vi "Test.vi"() -> ()   [LabVIEW 2018]
uses:
  controls/openModbusConnectionCluster.ctl
  controls/writeSingleRegisterModbusCluster.ctl
  controls/modbusDriverSelectorEnum.ctl
  controls/readRegisterModbusCluster.ctl
panel:
  in  "Register to write":u16
  in  "Address":u16
  in  "Write":bool
  out "Boolean":bool
  in  "Port":u16=255
  in  "Timeout":i32=500
  in  "IP Address":string
  in  "OK":bool
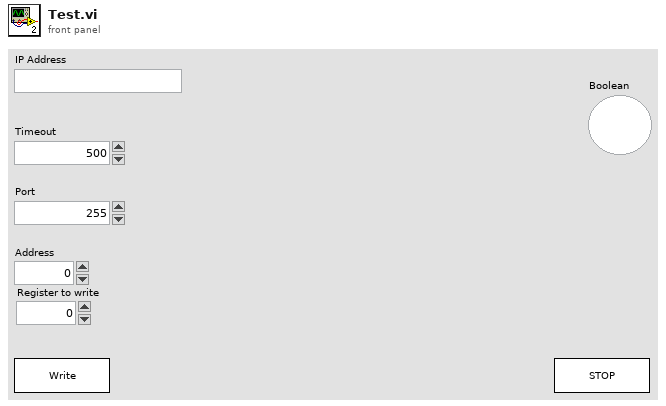
[diagram p1: front panel]
types:
  T1 = enum32{"Invalid", "Standard", "Closed", "Hidden", "Minimized", "Maximized"}
  T2 = enum32{"invalid app kind", "Development System", "Run Time System", "Student Edition", "Embedded LabVIEW", "Evaluation", "Custom"}
  T3 = typedef "writeSingleRegisterModbusCluster.ctl" = cluster{"Address":u16, "Register to write":u16}
  T4 = typedef "openModbusConnectionCluster.ctl" = cluster{"IP Address":string, "Timeout (ms)":i32, "Port (502)":u16}
  T5 = typedef "modbusDriverSelectorEnum.ctl" = enum16{"open", "write single holding registers", "read holding registers", "close"}
  T6 = typedef "readRegisterModbusCluster.ctl" = cluster{"Starting Address":u16, "Number of Inputs":u16}
  T7 = cluster{"Core":cluster{"Current VI Reference":refnum<vi>, "Close Panel on Exit?":bool}, "Open Modbus Connection Cluster":T4, bool, "Write Single Register Modbus":T3}
  T8 = cluster{"Current VI Reference":refnum<vi>, "Close Panel on Exit?":bool}
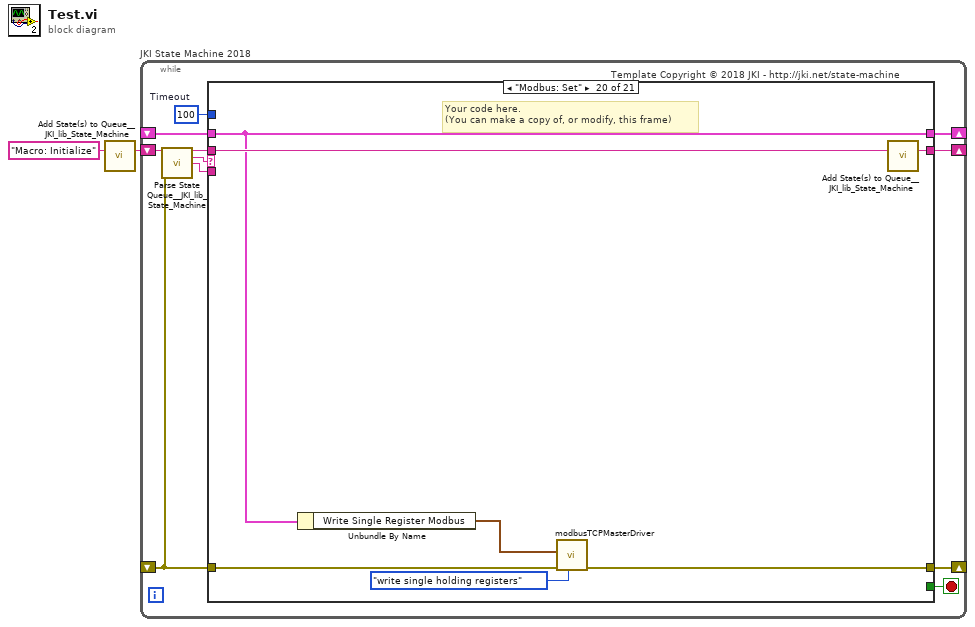
[diagram p0: block diagram]
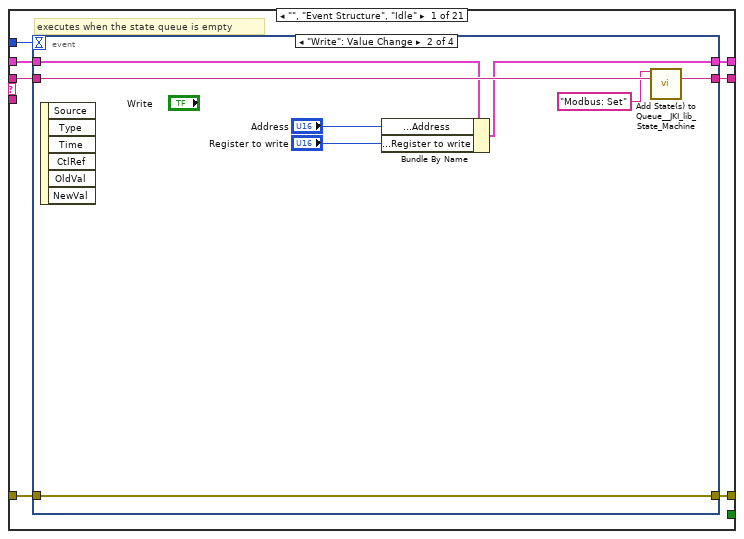
[diagram p2: hidden frame]
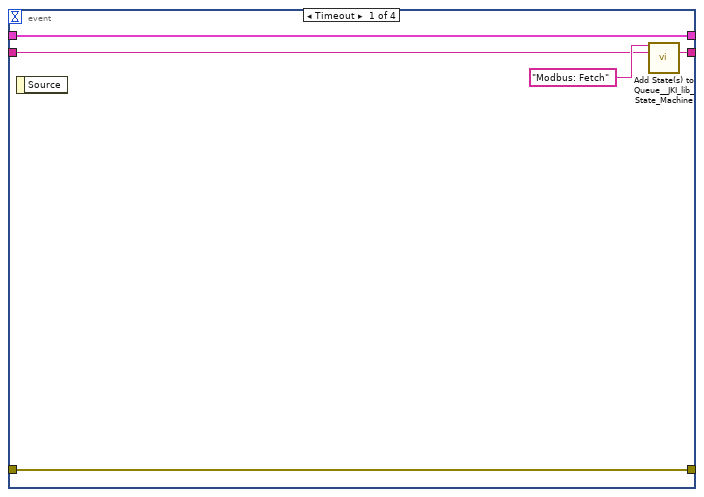
[diagram p3: hidden frame]
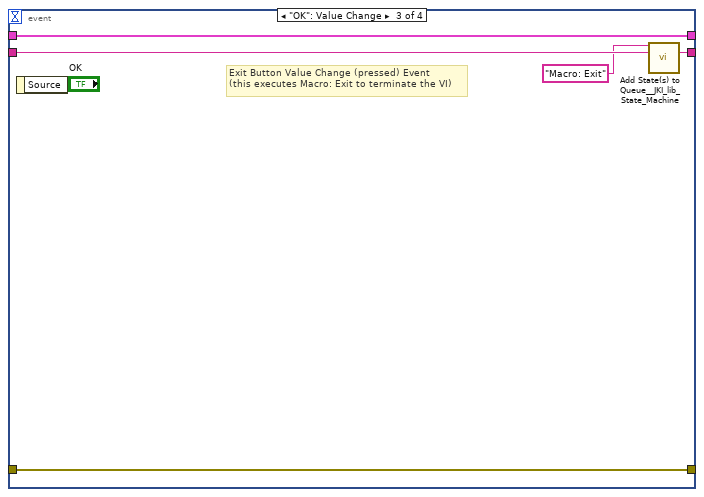
[diagram p4: hidden frame]
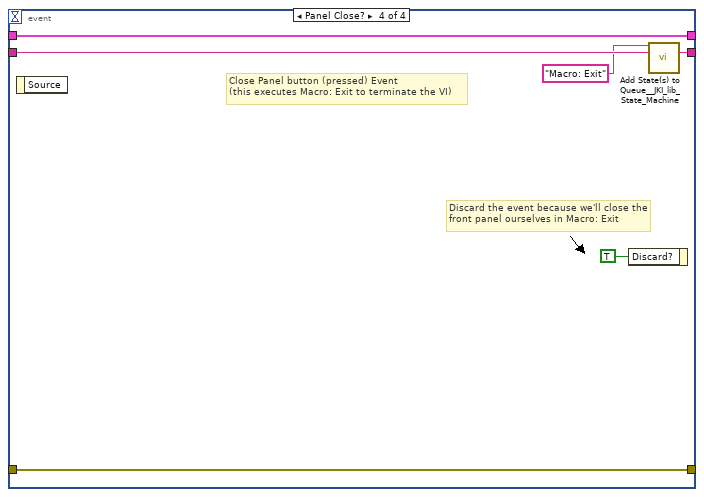
[diagram p5: hidden frame]
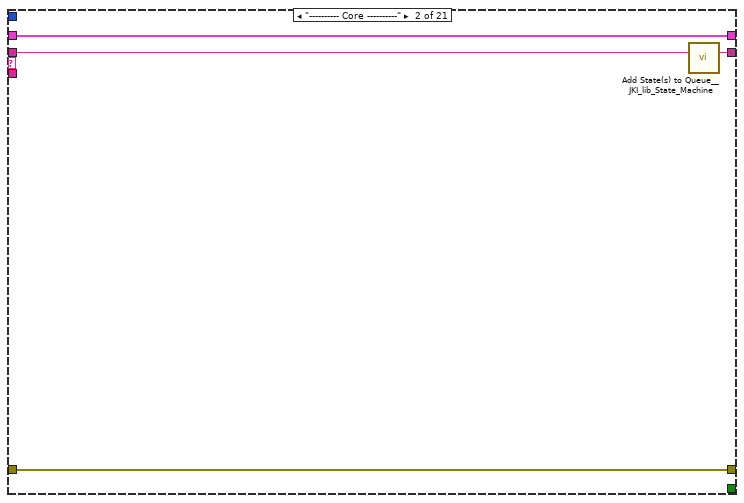
[diagram p6: hidden frame]
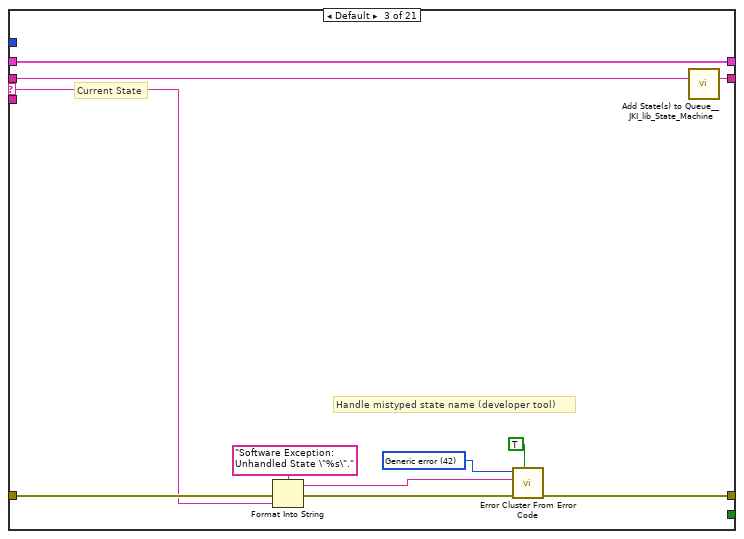
[diagram p7: hidden frame]
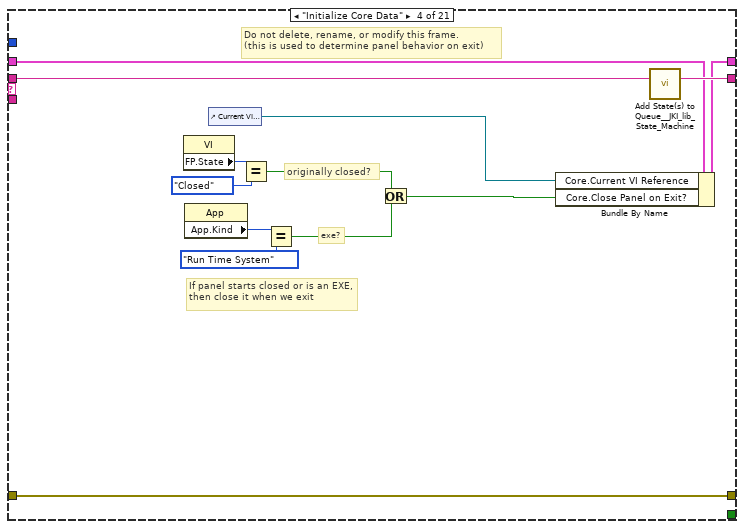
[diagram p8: hidden frame]
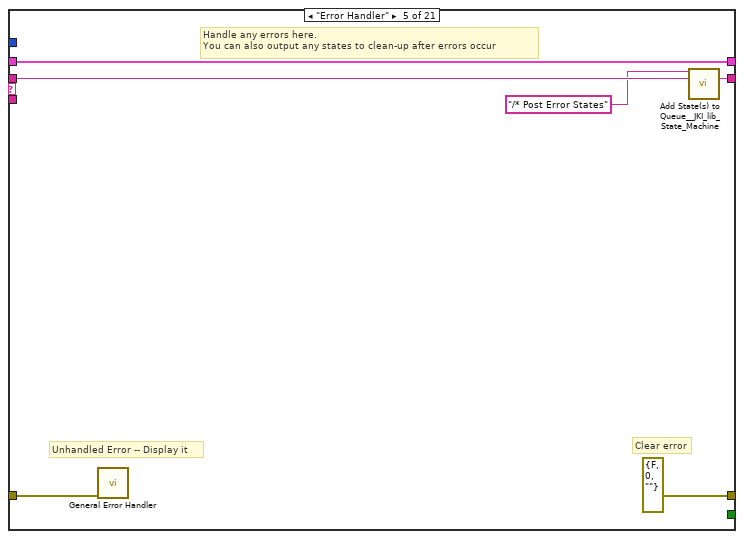
[diagram p9: hidden frame]
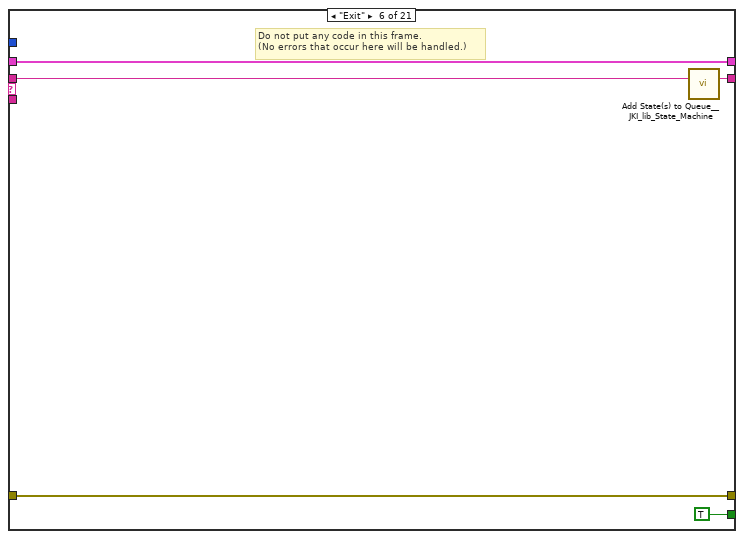
[diagram p10: hidden frame]
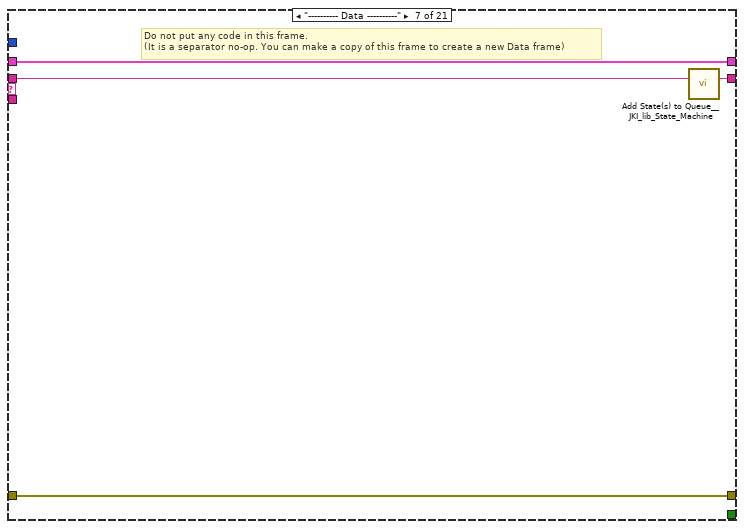
[diagram p11: hidden frame]
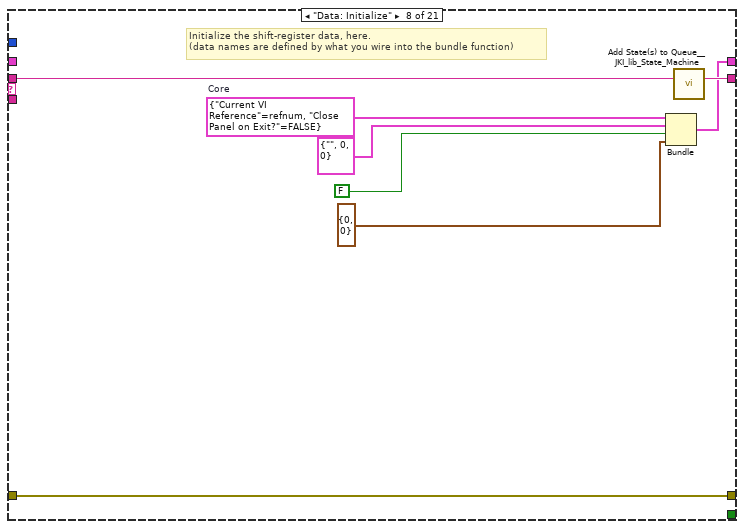
[diagram p12: hidden frame]
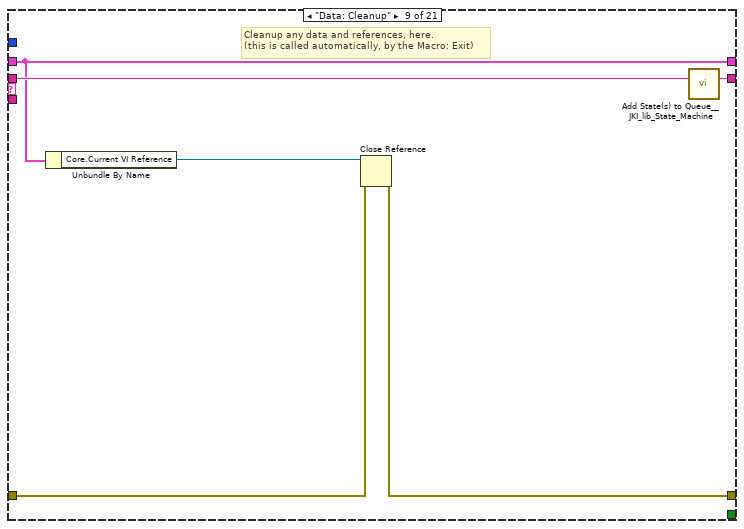
[diagram p13: hidden frame]
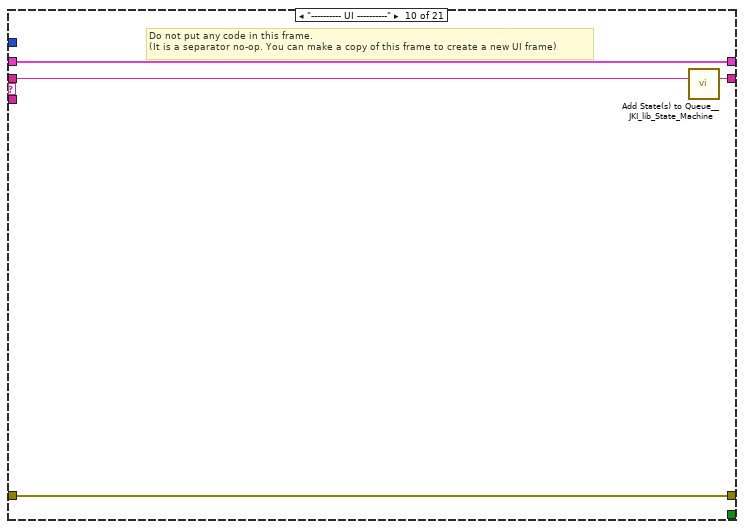
[diagram p14: hidden frame]
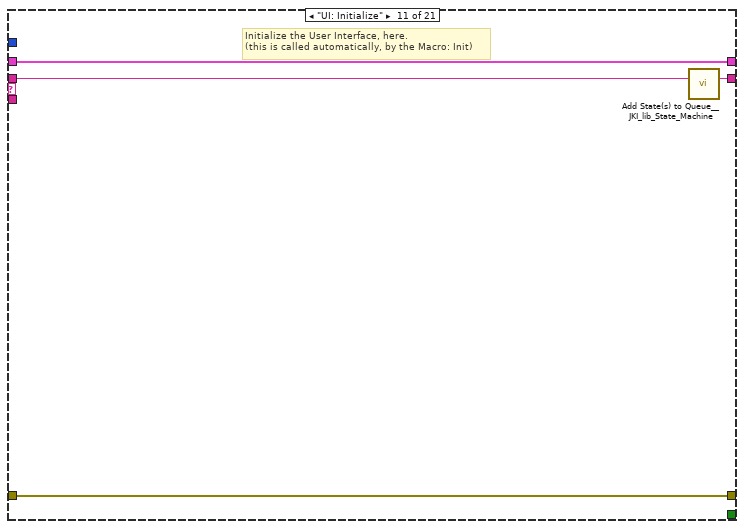
[diagram p15: hidden frame]
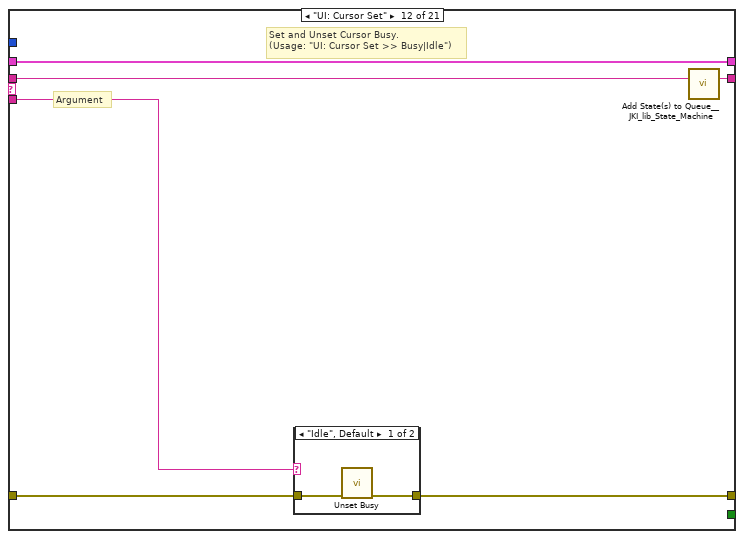
[diagram p16: hidden frame]
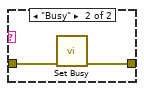
[diagram p17: hidden frame]
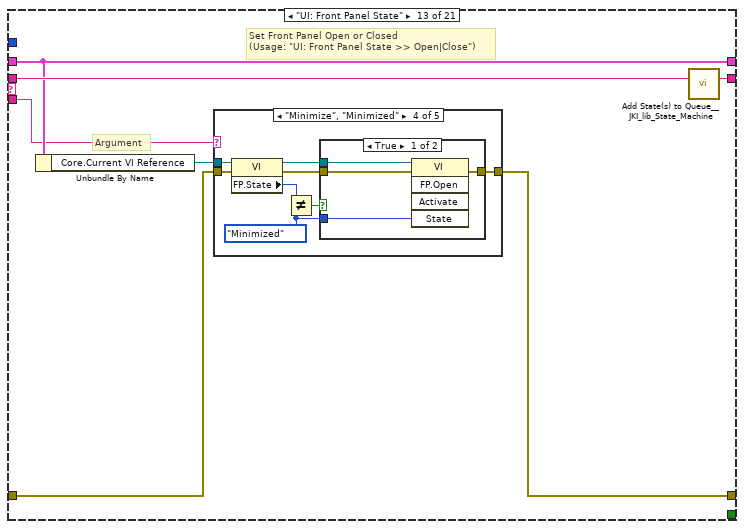
[diagram p18: hidden frame]
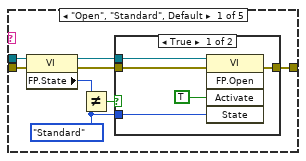
[diagram p19: hidden frame]
diagram:
  n1 = call <vilib>:"Add State(s) to Queue__JKI_lib_State_Machine.vi"("State(s) in (\"\")"="Macro: Initialize") -> ("States Out"=w2:string)  [unwired: 14 in]
  n2 = while "JKI State Machine 2018" {
    shift-right: [w6] -> _
    shift-left: _ -> [w5]
    shift-right: [w9] -> _
    shift-left: _ -> [w3]
    shift-right: [w8] -> _
    shift-left: w2 -> [w10]
    stop <- w7 stop-if-true
    w4 = 100  # Timeout
    # "Template Copyright © 2018 JKI - http://jki.net/state-machine"
    n3 = call <vilib>:"Parse State Queue__JKI_lib_State_Machine.vi"("State Queue"=w10, "Error In (no error)"=w3) -> ("Remaining States"=w12:string, "Current State"=w13:string, "Arguments"=w11:string)  [unwired: 11 in]
    n4 = case shown="\"Modbus: Set\"" w13 {
      selector: w13 -> [_ _ w49 _ _ _ _ _ _ _ _ _ _ _ _ _ _ _ _ _ _]
      tunnel: w12 -> [w20 w48 w53 w72 w78 w83 w87 w95 w101 w105 w109 w115 w126 w195 w200 w210 w214 w225 w239 w249 w253]
      tunnel: w11 -> [_ _ _ _ _ _ _ _ _ _ _ w110 w120 _ _ _ _ _ _ _ _]
      tunnel: w5 -> [w18 w45 w51 w65 w75 w81 w84 _ w96 w102 w107 w113 w122 w192 w197 w207 w211 w223 w237 w244 w250]
      tunnel: [w17 w46 w55 w69 errorcluster {"status"=FALSE, "code"=0, "source"=""} ("error out") w80 w85 w92 w97 w103 w106 w111 w123 w193 w198 w208 w212 w221 w235 w246 w251] -> w9
      tunnel: w3 -> [w16 w46 w54 w69 w74 w80 w85 w92 w98 w103 w106 w112 w124 w193 w198 w208 w212 w222 w236 w247 w251]
      tunnel: [w19 w47 w52 w71 w77 w82 w86 w94 w100 w104 w108 w114 w125 w194 w199 w209 w213 w224 w238 w248 w252] -> w8
      tunnel: [_ _ _ _ _ TRUE _ _ _ _ _ _ _ _ _ _ _ _ _ _ _] -> w7
      tunnel: [w15 w45 w51 w70 w75 w81 w84 w93 w96 w102 w107 w113 w122 w192 w197 w207 w211 w223 w237 w244 w250] -> w6
      tunnel: w4 -> [w14 _ _ _ _ _ _ _ _ _ _ _ _ _ _ _ _ _ _ _ _]
      frame "", "Event Structure", "Idle" {
        # "executes when the state queue is empty"
        n5 = event shown="[1] \"Write\": Value Change" {
          selector: _ -> [_ _ _ _]
          dyn-events: _ -> [_ _ _ _]
          timeout: w14 -> [_ _ _ _]
          tunnel: w20 -> [w21 w33 w38 w44]
          tunnel: [w25 w32 w37 w43] -> w19
          tunnel: w18 -> [w23 w30 w35 w41]
          tunnel: [w24 w27 w36 w42] -> w17
          tunnel: w16 -> [w24 w27 w36 w42]
          tunnel: [w23 w29 w35 w41] -> w15
          event Timeout {
            n6 = event-data() -> ()  [unwired: 1 in, 1 out]
            n7 = call <vilib>:"Add State(s) to Queue__JKI_lib_State_Machine.vi"("State(s) in Front (\"\")"="Modbus: Fetch", "State(s) in (\"\")"=w21) -> ("States Out"=w25:string)  [unwired: 13 in]
          }
          event "Write": Value Change {
            n8 = event-data() -> ()  [unwired: 1 in, 6 out]
            n9 = Bundle By Name(cluster=w30, "Write Single Register Modbus.Address"="Address", "Write Single Register Modbus.Register to write"="Register to write") -> (w29:T7)
            n10 = call <vilib>:"Add State(s) to Queue__JKI_lib_State_Machine.vi"("State(s) in Front (\"\")"="Modbus: Set" ("State(s) in Front (\"\")"), "State(s) in (\"\")"=w33) -> ("States Out"=w32:string)  [unwired: 13 in]
          }
          event "OK": Value Change {
            # "Exit Button Value Change (pressed) Event\n(this executes Macro: Exit to terminate the VI)"
            n11 = event-data() -> ()  [unwired: 1 in, 1 out]
            n12 = call <vilib>:"Add State(s) to Queue__JKI_lib_State_Machine.vi"("State(s) in Front (\"\")"="Macro: Exit", "State(s) in (\"\")"=w38) -> ("States Out"=w37:string)  [unwired: 13 in]
          }
          event Panel Close? {
            # "Discard the event because we'll close the front panel ourselves in Macro: Exit"
            # "Close Panel button (pressed) Event\n(this executes Macro: Exit to terminate the VI)"
            n13 = event-data() -> ()  [unwired: 1 in, 1 out]
            n14 = event-data("Discard?"=TRUE) -> ()  [unwired: 1 in, 1 out]
            n15 = call <vilib>:"Add State(s) to Queue__JKI_lib_State_Machine.vi"("State(s) in Front (\"\")"="Macro: Exit", "State(s) in (\"\")"=w44) -> ("States Out"=w43:string)  [unwired: 13 in]
          }
        }
      }
      frame "---------- Core ----------" {
        n16 = call <vilib>:"Add State(s) to Queue__JKI_lib_State_Machine.vi"("State(s) in (\"\")"=w48) -> ("States Out"=w47:string)  [unwired: 14 in]
      }
      frame Default {
        w58 = 42 items=["No error", "Argument error", "Memory is full", "Out of zone", "End of file", "File already open", "Generic file I/O error", "File not found", "File permission error", "Disk is full", "Duplicate path", "Too many files open", "System feature not enabled", "Resource file not found", "Cannot add resource", "Resource not found", "Image not found", "Image memory error", "Pen does not exist", "Config type invalid", "Config token not found", "Config parse error", "Config memory error", "Bad external code format", "Bad external code offset", "External code not present", "Null window", "Destroy window error", "Null menu", "Print aborted", "Bad print record", "Print driver error", "Windows error during printing", "Memory error during printing", "Print dialog error", "Generic print error", "Invalid device refnum", "Device not found", "Device parameter error", "Device unit error", "Cannot open device", "Device call aborted", "Generic error", "Cancelled by user", "Object ID too low", "Object ID too high", "Object not in heap", "Unknown heap", "Unknown object (invalid DefProc)", "Unknown object (DefProc not in table)", "Message out of range", "Invalid (null) method", "Unknown message", "Manager call not supported", "Bad address", "Network operation in progress", "Network operation timed out", "Connection is busy", "Network attribute not supported", "Network error", "Address in use", "System out of memory", "Connection aborted", "Connection refused", "Not connected", "Already connected", "Connection closed", "Initialization error (interapplication manager)", "Bad occurrence", "Wait on unbound occurrence handler", "Occurrence queue overflow", "Datalog type conflict", "Unused", "Unrecognized type (interapplication manager)", "Memory corrupt", "Failed to make temporary DLL", "Old CIN version", "Drag socket not found", "Failed to load drop-object", "Failed to register OLE object", "Failed to release OLE object", "Format specifier type mismatch", "Unknown format specifier", "Too few format specifiers", "Too many format specifiers", "Scan failed", "Newer CIN version", "Error converting to variant", "Runtime menu error", "Password tampered", "Variant attribute not found", "Incompatible variant data type", "Event data is not available", "Event Store is not present", "Occurrence is not found", "Event Queue is not created", "Event info is not available", "Refnum passed is NULL", "Error retrieving Class GUID", "Error retrieving CoClass GUID", "Error retrieving TypeLib GUID.", "Bad built application magic bytes.", "Specific driver is different from the specific driver associated with the Logical Name.", "There is no session opened to the class driver.", "Max Error", "MAX - Error with config objects", "MAX - Error loading configuration", "MAX - Group not supported"]
        # "Current State"
        # "Handle mistyped state name (developer tool)"
        n17 = Format Into String(format string="Software Exception: Unhandled State \"%s\"." ("message"), error in=w54, w49) -> (resulting string=w57:string, error out=w56:errorcluster)  [unwired: 1 in]
        n18 = call <vilib>:"Error Cluster From Error Code.vi"("show call chain? (False)"=TRUE, "error in (no error)"=w56, "error message (\"\")"=w57, "error code (0)"=w58) -> ("error out"=w55:errorcluster)  [unwired: 5 in]
        n19 = call <vilib>:"Add State(s) to Queue__JKI_lib_State_Machine.vi"("State(s) in (\"\")"=w53) -> ("States Out"=w52:string)  [unwired: 14 in]
      }
      frame "Initialize Core Data" {
        # "Do not delete, rename, or modify this frame.\n(this is used to determine panel behavior on exit)"
        # "originally closed?"
        # "exe?"
        # "If panel starts closed or is an EXE, then close it when we exit"
        n20 = property class="VI"() -> ("FP.State"=w62:T1)  [unwired: 2 in, 2 out]
        n21 = property class="App"() -> ("App.Kind"=w68:T2)  [unwired: 2 in, 2 out]
        n22 = control-ref of="Current VI Reference"() -> (w63:refnum<vi>)
        n23 = Equal?(x=w62, y=T1."Closed" ("Front Panel Window:State")) -> (x = y?=w60:bool)
        n24 = Equal?(x=w68, y=T2."Run Time System" ("Application:Kind")) -> (x = y?=w66:bool)
        n25 = Or(x=w60, y=w66) -> (x .or. y?=w64:bool)
        n26 = Bundle By Name(cluster=w65, "Core.Current VI Reference"=w63, "Core.Close Panel on Exit?"=w64) -> (w70:T7)
        n27 = call <vilib>:"Add State(s) to Queue__JKI_lib_State_Machine.vi"("State(s) in (\"\")"=w72) -> ("States Out"=w71:string)  [unwired: 14 in]
      }
      frame "Error Handler" {
        # "Unhandled Error -- Display it"
        # "Handle any errors here.\nYou can also output any states to clean-up after errors occur"
        # "Clear error"
        n28 = call <vilib>:"General Error Handler.vi"("error in (no error)"=w74) -> ()  [unwired: 10 in, 5 out]
        n29 = call <vilib>:"Add State(s) to Queue__JKI_lib_State_Machine.vi"("State(s) in Front (\"\")"="/* Post Error States", "State(s) in (\"\")"=w78) -> ("States Out"=w77:string)  [unwired: 13 in]
      }
      frame "Exit" {
        # "Do not put any code in this frame.\n(No errors that occur here will be handled.)"
        n30 = call <vilib>:"Add State(s) to Queue__JKI_lib_State_Machine.vi"("State(s) in (\"\")"=w83) -> ("States Out"=w82:string)  [unwired: 14 in]
      }
      frame "---------- Data ----------" {
        # "Do not put any code in this frame.\n(It is a separator no-op. You can make a copy of this frame to create a new Data frame)"
        n31 = call <vilib>:"Add State(s) to Queue__JKI_lib_State_Machine.vi"("State(s) in (\"\")"=w87) -> ("States Out"=w86:string)  [unwired: 14 in]
      }
      frame "Data: Initialize" {
        w91 = T8 {"Current VI Reference"=refnum, "Close Panel on Exit?"=FALSE}  # Core
        # "Initialize the shift-register data, here.\n(data names are defined by what you wire into the bundle function)"
        n32 = Bundle("Core"=w91, "Open Modbus Connection Cluster"=T4 {"IP Address"="", "Timeout (ms)"=0, "Port (502)"=0}, FALSE, "Write Single Register Modbus"=T3 {"Address"=0, "Register to write"=0}) -> (w93:T7)  [unwired: 1 in]
        n33 = call <vilib>:"Add State(s) to Queue__JKI_lib_State_Machine.vi"("State(s) in (\"\")"=w95) -> ("States Out"=w94:string)  [unwired: 14 in]
      }
      frame "Data: Cleanup" {
        # "Cleanup any data and references, here.\n(this is called automatically, by the Macro: Exit)"
        n34 = Unbundle By Name(w96) -> ("Core.Current VI Reference"=w99:refnum<vi>)
        n35 = Close Reference(reference=w99, error in (no error)=w98) -> (error out=w97:errorcluster)
        n36 = call <vilib>:"Add State(s) to Queue__JKI_lib_State_Machine.vi"("State(s) in (\"\")"=w101) -> ("States Out"=w100:string)  [unwired: 14 in]
      }
      frame "---------- UI ----------" {
        # "Do not put any code in this frame.\n(It is a separator no-op. You can make a copy of this frame to create a new UI frame)"
        n37 = call <vilib>:"Add State(s) to Queue__JKI_lib_State_Machine.vi"("State(s) in (\"\")"=w105) -> ("States Out"=w104:string)  [unwired: 14 in]
      }
      frame "UI: Initialize" {
        # "Initialize the User Interface, here.\n(this is called automatically, by the Macro: Init)"
        n38 = call <vilib>:"Add State(s) to Queue__JKI_lib_State_Machine.vi"("State(s) in (\"\")"=w109) -> ("States Out"=w108:string)  [unwired: 14 in]
      }
      frame "UI: Cursor Set" {
        # "Argument"
        # "Set and Unset Cursor Busy.\n(Usage: \"UI: Cursor Set >> Busy|Idle\")"
        n39 = case shown="\"Idle\", Default" w110 {
          tunnel: w112 -> [w117 w119]
          tunnel: [w116 w118] -> w111
          frame "Idle", Default {
            n40 = call <vilib>:"Unset Busy.vi"("error in (no error)"=w117) -> ("error out"=w116:errorcluster)  [unwired: 10 in]
          }
          frame "Busy" {
            n41 = call <vilib>:"Set Busy.vi"("error in (no error)"=w119) -> ("error out"=w118:errorcluster)  [unwired: 9 in, 1 out]
          }
        }
        n42 = call <vilib>:"Add State(s) to Queue__JKI_lib_State_Machine.vi"("State(s) in (\"\")"=w115) -> ("States Out"=w114:string)  [unwired: 14 in]
      }
      frame "UI: Front Panel State" {
        # "Argument"
        # "Set Front Panel Open or Closed\n(Usage: \"UI: Front Panel State >> Open|Close\")"
        n43 = Unbundle By Name(w122) -> ("Core.Current VI Reference"=w121:refnum<vi>)
        n44 = case shown="\"Minimize\", \"Minimized\"" w120 {
          tunnel: w124 -> [w132 w147 w158 w171 w184]
          tunnel: [w134 w148 w160 w173 w186] -> w123
          tunnel: w121 -> [w133 w145 w159 w172 w185]
          frame "Open", "Standard", Default {
            w127 = T1."Standard" ("State")
            n45 = property class="VI"(reference=w133, error in=w132) -> (reference out=w130:refnum<vi>, error out=w131:errorcluster, "FP.State"=w129:T1)
            n46 = Not Equal?(x=w129, y=w127) -> (x != y?=w128:bool)
            n47 = case shown="True" w128 {
              tunnel: [w138 w140] -> w134
              tunnel: w131 -> [w137 w140]
              tunnel: w130 -> [w136 _]
              tunnel: w127 -> [w135 _]
              frame True {
                n48 = invoke class="VI" method="FP.Open"(reference=w136, error in=w137, "Activate"=TRUE, "State"=w135) -> (error out=w138:errorcluster)  [unwired: 1 in, 4 out]
              }
              frame False {
              }
            }
          }
          frame "Close", "Closed" {
            n49 = property class="VI"(reference=w145, error in=w147) -> (reference out=w144:refnum<vi>, error out=w146:errorcluster, "FP.State"=w142:T1)
            n50 = Not Equal?(x=w142, y=T1."Closed" ("Front Panel Window:State")) -> (x != y?=w141:bool)
            n51 = case shown="True" w141 {
              tunnel: [w149 w152] -> w148
              tunnel: w146 -> [w149 w151]
              tunnel: w144 -> [_ w150]
              frame False {
              }
              frame True {
                n52 = invoke class="VI" method="FP.Close"(reference=w150, error in=w151) -> (error out=w152:errorcluster)  [unwired: 1 in, 2 out]
              }
            }
          }
          frame "Hidden", "Hide" {
            w153 = T1."Hidden" ("State")
            n53 = property class="VI"(reference=w159, error in=w158) -> (reference out=w156:refnum<vi>, error out=w157:errorcluster, "FP.State"=w155:T1)
            n54 = Not Equal?(x=w155, y=w153) -> (x != y?=w154:bool)
            n55 = case shown="True" w154 {
              tunnel: [w164 w165] -> w160
              tunnel: w157 -> [w163 w165]
              tunnel: w156 -> [w162 _]
              tunnel: w153 -> [w161 _]
              frame True {
                n56 = invoke class="VI" method="FP.Open"(reference=w162, error in=w163, "State"=w161) -> (error out=w164:errorcluster)  [unwired: 2 in, 4 out]
              }
              frame False {
              }
            }
          }
          frame "Minimize", "Minimized" {
            w166 = T1."Minimized" ("State")
            n57 = property class="VI"(reference=w172, error in=w171) -> (reference out=w169:refnum<vi>, error out=w170:errorcluster, "FP.State"=w168:T1)
            n58 = Not Equal?(x=w168, y=w166) -> (x != y?=w167:bool)
            n59 = case shown="True" w167 {
              tunnel: [w177 w178] -> w173
              tunnel: w170 -> [w176 w178]
              tunnel: w169 -> [w175 _]
              tunnel: w166 -> [w174 _]
              frame True {
                n60 = invoke class="VI" method="FP.Open"(reference=w175, error in=w176, "State"=w174) -> (error out=w177:errorcluster)  [unwired: 2 in, 4 out]
              }
              frame False {
              }
            }
          }
          frame "Maximize", "Maximized" {
            w179 = T1."Maximized" ("State")
            n61 = property class="VI"(reference=w185, error in=w184) -> (reference out=w182:refnum<vi>, error out=w183:errorcluster, "FP.State"=w181:T1)
            n62 = Not Equal?(x=w181, y=w179) -> (x != y?=w180:bool)
            n63 = case shown="True" w180 {
              tunnel: [w190 w191] -> w186
              tunnel: w183 -> [w189 w191]
              tunnel: w182 -> [w188 _]
              tunnel: w179 -> [w187 _]
              frame True {
                n64 = invoke class="VI" method="FP.Open"(reference=w188, error in=w189, "State"=w187) -> (error out=w190:errorcluster)  [unwired: 2 in, 4 out]
              }
              frame False {
              }
            }
          }
        }
        n65 = call <vilib>:"Add State(s) to Queue__JKI_lib_State_Machine.vi"("State(s) in (\"\")"=w126) -> ("States Out"=w125:string)  [unwired: 14 in]
      }
      frame "---------- Macro ----------" {
        # "Do not put any code in this frame.\n(It is a separator no-op. You can make a copy of this frame to create a new Macro frame)"
        n66 = call <vilib>:"Add State(s) to Queue__JKI_lib_State_Machine.vi"("State(s) in (\"\")"=w195) -> ("States Out"=w194:string)  [unwired: 14 in]
      }
      frame "Macro: Initialize" {
        w196 = "Data: Initialize\nInitialize Core Data\nUI: Initialize\nUI: Front Panel State >> Open\nModbus: Init"  # Data: Initialize Initialize Core Data UI: Initialize UI: Front Panel State >> Open Modbus: Init
        # "Initialization Macro\n(This is called once, when the VI starts)"
        n67 = call <vilib>:"Add State(s) to Queue__JKI_lib_State_Machine.vi"("State(s) in Front (\"\")"=w196, "State(s) in (\"\")"=w200) -> ("States Out"=w199:string)  [unwired: 13 in]
      }
      frame "Macro: Exit" {
        # "Exit Macro\n(This is called once, when the VI exits)"
        n68 = Unbundle By Name(w207) -> ("Core.Close Panel on Exit?"=w206:bool)
        n69 = Select(t="UI: Front Panel State >> Close", s=w206, f="") -> (s? t:f=w203:string)
        n70 = call <vilib>:"Add State(s) to Queue__JKI_lib_State_Machine.vi"("State(s) in (\"\")"=w203, "State(s) at Back (\"\")"="Modbus: Close\nData: Cleanup\nExit") -> ("States Out"=w201:string)  [unwired: 13 in]
        n71 = call <vilib>:"Add State(s) to Queue__JKI_lib_State_Machine.vi"("State(s) in Front (\"\")"=w201, "State(s) in (\"\")"=w210) -> ("States Out"=w209:string)  [unwired: 13 in]
      }
      frame "---------- Modbus ----------" {
        # "Template Separator\n(You can make a copy of, or modify, this frame)"
        n72 = call <vilib>:"Add State(s) to Queue__JKI_lib_State_Machine.vi"("State(s) in (\"\")"=w214) -> ("States Out"=w213:string)  [unwired: 14 in]
      }
      frame "Modbus: Init" {
        # "Your code here.\n(You can make a copy of, or modify, this frame)"
        n73 = Bundle By Name(cluster=T4 {"IP Address"="", "Timeout (ms)"=0, "Port (502)"=0} ("Open Modbus Connection Cluster"), "IP Address"="IP Address", "Timeout (ms)"="Timeout", "Port (502)"="Port") -> (w218:T4)
        n74 = call "modbusTCPMasterDriver.vi"("Modbus Driver Selector Enum"=modbusDriverSelectorEnum."open", "Error In"=w222, "Open Modbus Connection Cluster"=w218) -> ("Error Out"=w221:errorcluster)  [unwired: 7 in, 1 out]
        n75 = call <vilib>:"Add State(s) to Queue__JKI_lib_State_Machine.vi"("State(s) in (\"\")"=w225) -> ("States Out"=w224:string)  [unwired: 14 in]
      }
      frame "Modbus: Fetch" {
        # "Your code here.\n(You can make a copy of, or modify, this frame)"
        n76 = call "modbusTCPMasterDriver.vi"("Modbus Driver Selector Enum"=modbusDriverSelectorEnum."read holding registers", "Error In"=w236, "Read Modbus Register"=T6 {"Starting Address"=0, "Number of Inputs"=1}) -> ("Error Out"=w235:errorcluster, "Register Value"=w232:u16[])  [unwired: 7 in]
        n77 = Index Array(array=w232, index=0) -> (element=w230:u16)
        n78 = Equal?(x=w230, y=u16 1) -> (x = y?=w228:bool)
        n79 = feedback-in #1(w228) -> ()
        n80 = feedback #1() -> (w227:bool)  [unwired: 1 in]
        n81 = case shown="False" w227 {
          selector: w227 -> [_ w241]
          tunnel: ["" "Modbus: Set"] -> w226
          frame False {
          }
          frame True {
            "Boolean" <- w241
          }
        }
        n82 = call <vilib>:"Add State(s) to Queue__JKI_lib_State_Machine.vi"("State(s) in Front (\"\")"=w226, "State(s) in (\"\")"=w239) -> ("States Out"=w238:string)  [unwired: 13 in]
      }
      frame "Modbus: Set" {
        # "Your code here.\n(You can make a copy of, or modify, this frame)"
        n83 = Unbundle By Name(w244) -> ("Write Single Register Modbus"=w243:T3)
        n84 = call "modbusTCPMasterDriver.vi"("Modbus Driver Selector Enum"=modbusDriverSelectorEnum."write single holding registers", "Error In"=w247, "Write Single Register Modbus"=w243) -> ("Error Out"=w246:errorcluster)  [unwired: 7 in, 1 out]
        n85 = call <vilib>:"Add State(s) to Queue__JKI_lib_State_Machine.vi"("State(s) in (\"\")"=w249) -> ("States Out"=w248:string)  [unwired: 14 in]
      }
      frame "Modbus: Close" {
        # "Your code here.\n(You can make a copy of, or modify, this frame)"
        n86 = call <vilib>:"Add State(s) to Queue__JKI_lib_State_Machine.vi"("State(s) in (\"\")"=w253) -> ("States Out"=w252:string)  [unwired: 14 in]
      }
    }
  }
